vi "Destroy_Events.vi"(8 "error in (no error)":errorcluster, 11 "Test_Nested in":refnum<class "Test_Nested.lvclass">) -> (0 "error out":errorcluster, 3 "Test_Nested out":refnum<class "Test_Nested.lvclass">)   [LabVIEW 2025, in "Test_Nested.lvlib" / "Test_Nested.lvclass"]
uses:
  Test_Nested.lvclass
  Test_Nested.lvclass/Test_Nested.ctl
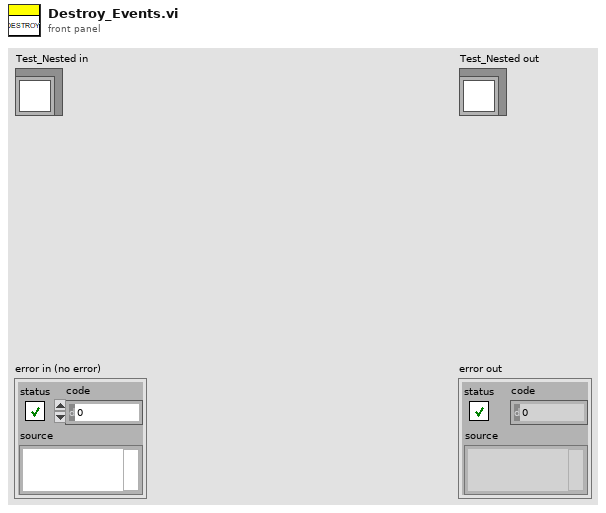
[diagram p1: front panel]
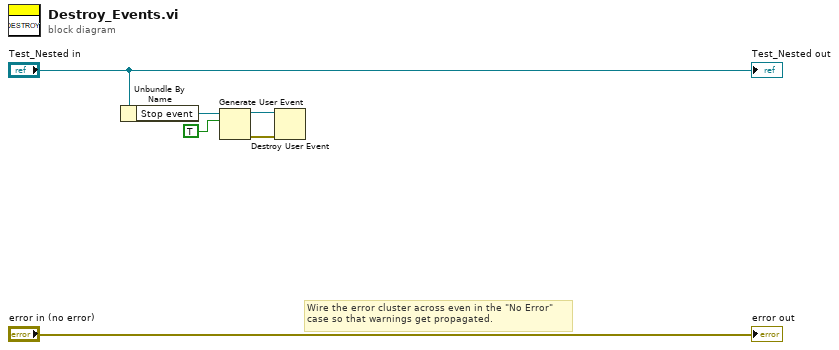
[diagram p0: block diagram]
diagram:
  # "Wire the error cluster across even in the \"No Error\"\ncase so that warnings get propagated."
  n1 = Unbundle By Name("Test_Nested in") -> ("Stop event"=w4:refnum<user-event>)
  n2 = Generate User Event(user event=w4, event data cluster=TRUE ("event data")) -> (user event out=w1:refnum<user-event>, error out=w2:errorcluster)  [unwired: 2 in]
  n3 = Destroy User Event(user event=w1, error in=w2) -> ()  [unwired: 1 out]
  "error out" <- "error in (no error)"
  "Test_Nested out" <- "Test_Nested in"
